vi "Всплывающий график.vi"(0 "Массив Y":dbl[](array[numeric]) format="%.2f", 1 "Массив X":dbl[](array[numeric]) format="%.2f") -> ()   [LabVIEW 2017]
doc: "This VI is an exercise in the LabVIEW Basics I course.\n\nThis VI displays X and Y data in a graph until the user presses the Done button. You will modify the VI Setup to make this VI open when called and close afterwards."
panel:
  in  "Done":bool
  out "XY Graph":cluster{"X Array":dbl[], "Y Array":dbl[]}(graph)
  # "*массивы цифровых\n элементов управления *"
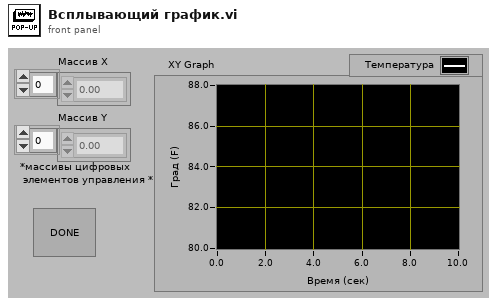
[diagram p1: front panel]
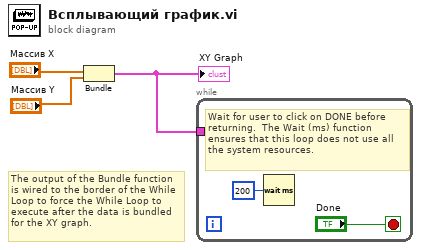
[diagram p0: block diagram]
diagram:
  # "The output of the Bundle function\nis wired to the border of the While Loop to force the While Loop to execute after the data is bundled\nfor the XY graph."
  n1 = Bundle("Массив X"="Массив X", "Массив Y"="Массив Y") -> (w1:cluster{"Массив X":dbl[], "Массив Y":dbl[]})  [unwired: 1 in]
  "XY Graph" <- w1
  n2 = while {
    tunnel: w1 -> [_]
    stop <- "Done" stop-if-true
    # "Wait for user to click on DONE before \nreturning.  The Wait (ms) function \nensures that this loop does not use all\nthe system resources."
    n3 = Wait (ms)(milliseconds to wait=u32 200) -> ()  [unwired: 1 out]
  }
